vi "libssh2_sftp_readdir_ex.vi"(5 "longentry maxlen (0)":i32, 7 "buffer maxlen":i32, 8 "error in (no error)":errorcluster, 11 "sftp handle":T2) -> (0 "error out":errorcluster, 1 "attrs":T1, 2 "buffer":string, 3 "no more files":bool, 4 "longentry":string)   [LabVIEW 2017, in "libssh2.lvlib"]
doc: "Read the next entry from a directory handle. Optionally return the output of a directory listing command."
uses:
  libssh2.lvlib
  SFTP Handle Refnum.ctl
  libssh2_sftp_attributes.ctl
  Acquire SFTP.vi
  Release SFTP.vi
  Acquire Session.vi
  Release Session.vi
  Not An SFTP Handle Refnum.vi
  <vilib>/Utility/error.llb/Error Cluster From Error Code.vi
  Global Settings.vi
  Read SFTP Handle Refnum.vi
  Read SFTP Refnum.vi
  Read Session Refnum.vi
  <vilib>/Utility/semaphor.llb/Acquire Semaphore.vi
  <vilib>/Utility/semaphor.llb/Release Semaphore.vi
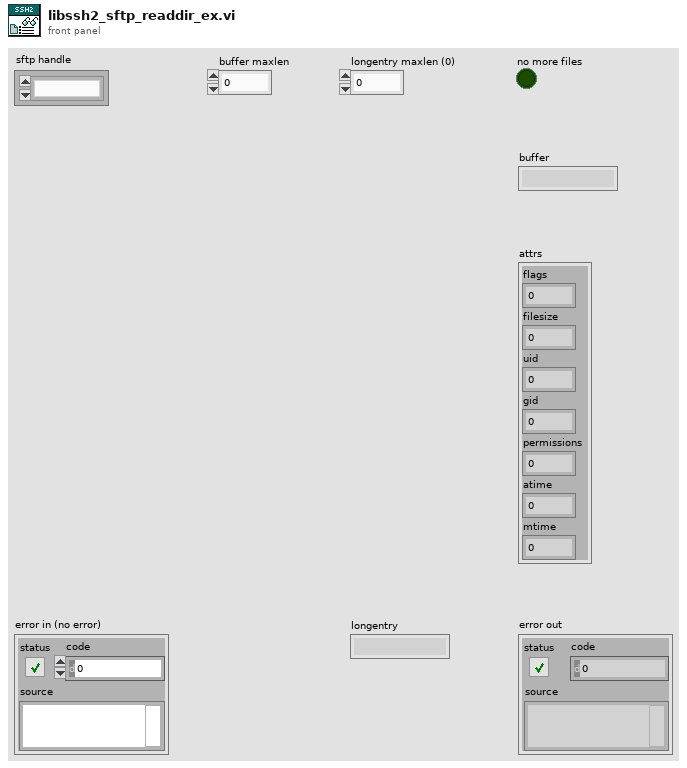
[diagram p1: front panel]
types:
  T1 = typedef "libssh2.lvlib/libssh2_sftp_attributes.ctl" = cluster{"flags":u32, "filesize":u64, "uid":u32, "gid":u32, "permissions":u32, "atime":u32, "mtime":u32}
  T2 = typedef "libssh2.lvlib/SFTP Handle Refnum.ctl" = refnum<k1>
  T3 = cluster{"flags":u32, "<padding1>":u32, "filesize":u64, "uid":u32, "gid":u32, "permissions":u32, "atime":u32, "mtime":u32, "<padding2>":u32}
  T4 = cluster{"flags":u32, "<padding1>":u32, "filesize":u64, "uid":u32, "<padding2>":u32, "gid":u32, "<padding3>":u32, "permissions":u32, "<padding4>":u32, "atime":u32, "<padding5>":u32, "mtime":u32, "<padding6>":u32}
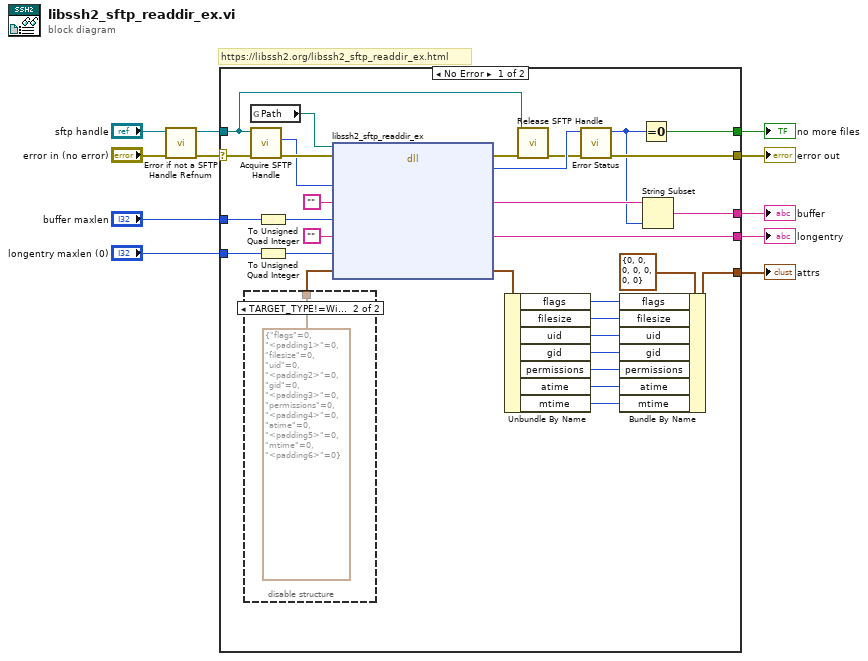
[diagram p0: block diagram]
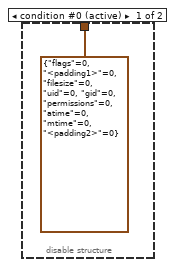
[diagram p2: hidden frame]
diagram:
  # "https://libssh2.org/libssh2_sftp_readdir_ex.html"
  n1 = call "Error if not a SFTP Handle Refnum.vi"("error in (no error)"="error in (no error)", "sftp handle"="sftp handle") -> ("error out"=w10:errorcluster, "sftp handle out"=w9:T2)  [unwired: 8 in]
  n2 = case shown="No Error" w10 {
    selector: w10 -> [w41 w45]
    tunnel: w9 -> [w12 _]
    tunnel: [w37 w45] -> w8
    tunnel: "buffer maxlen" -> [w35 _]
    tunnel: "longentry maxlen (0)" -> [w34 _]
    tunnel: [w30 _] -> w4
    tunnel: [w29 _] -> w3
    tunnel: [w14 _] -> w1
    tunnel: [w27 _] -> w2
    frame No Error {
      n3 = disable-structure shown="TARGET_TYPE!=Windows&&TARGET_BITNESS==64" {
        disable-tunnel: [T3 {"flags"=0, "<padding1>"=0, "filesize"=0, "uid"=0, "gid"=0, "permissions"=0, "atime"=0, "mtime"=0, "<padding2>"=0} ("attrs") T4 {"flags"=0, "<padding1>"=0, "filesize"=0, "uid"=0, "<padding2>"=0, "gid"=0, "<padding3>"=0, "permissions"=0, "<padding4>"=0, "atime"=0, "<padding5>"=0, "mtime"=0, "<padding6>"=0} ("attrs")] -> w24
        frame condition #0 (active) {
        }
        frame condition #1 {
        }
      }
      n4 = global read "Global Settings.vi" "Path"() -> (w42:path)
      n5 = call "Acquire SFTP Handle.vi"("error in (no error)"=w41, "sftp handle"=w12) -> ("error out"=w40:errorcluster, "LIBSSH2_SFTP_HANDLE*"=w39:u64)  [unwired: 8 in]
      n6 = To Unsigned Quad Integer(1:w35) -> (0:w32:u64)
      n7 = To Unsigned Quad Integer(1:w34) -> (0:w33:u64)
      n8 = dll-call lib="?" fn="libssh2_sftp_readdir_ex"(path in=w42, error in=w40, "handle"=w39, "buffer"="", "buffer_maxlen"=w32, "longentry"="", "longentry_maxlen"=w33, "attrs"=w24) -> (error out=w38:errorcluster, "return value"=w36:i32, "buffer"=w31:string, "longentry"=w29:string, "attrs"=w23:T3)  [unwired: 4 in, 1 out]
      n9 = Unbundle By Name(w23) -> ("flags"=w21:u32, "filesize"=w20:u64, "uid"=w19:u32, "gid"=w18:u32, "permissions"=w17:u32, "atime"=w16:u32, "mtime"=w15:u32)
      n10 = call "Release SFTP Handle.vi"("error in (no error)"=w38, "sftp handle"=w12) -> ("error out"=w13:errorcluster)  [unwired: 9 in]
      n11 = call "Error Status.vi"("error in (no error)"=w13, "return value"=w36) -> ("error out"=w37:errorcluster, "return value out"=w28:i32)  [unwired: 8 in]
      n12 = Bundle By Name(cluster=T1 {"flags"=0, "filesize"=0, "uid"=0, "gid"=0, "permissions"=0, "atime"=0, "mtime"=0} ("attrs"), "flags"=w21, "filesize"=w20, "uid"=w19, "gid"=w18, "permissions"=w17, "atime"=w16, "mtime"=w15) -> (w14:T1)
      n13 = Equal To 0?(x=w28) -> (x = 0?=w27:bool)
      n14 = String Subset(string=w31, length (rest)=w28) -> (substring=w30:string)  [unwired: 1 in]
    }
    frame Error {
    }
  }
  "error out" <- w8
  "buffer" <- w4
  "longentry" <- w3
  "attrs" <- w1
  "no more files" <- w2
